vi "Graphics-Init X-axis Overlay.vi"(0 "Ctl Refnum":refnum<vi>, 7 "X-axis slider":refnum<vi>, 11 "error in (no error)":errorcluster) -> (15 "error out":errorcluster)   [LabVIEW 2020]
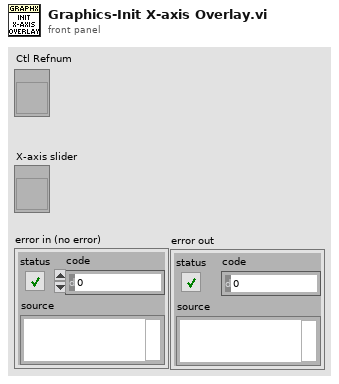
[diagram p1: front panel]
types:
  T1 = typedef "LVRectTypeDef.ctl" = cluster{"Left":i16, "Top":i16, "Right":i16, "Bottom":i16}
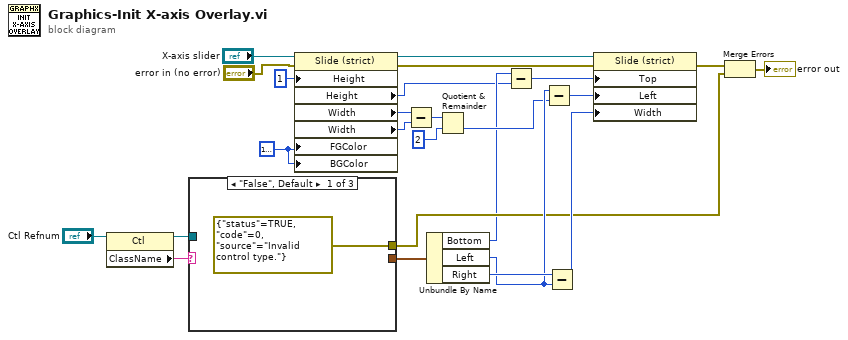
[diagram p0: block diagram]
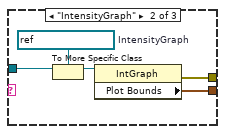
[diagram p2: hidden frame]
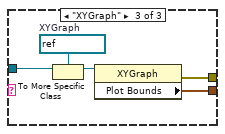
[diagram p3: hidden frame]
diagram:
  w8 = u32 16777216
  n1 = property class="Ctl"(reference="Ctl Refnum") -> (reference out=w5:refnum<vi>, "ClassName"=w6:string)  [unwired: 1 in, 1 out]
  n2 = case shown="\"False\", Default" w6 {
    tunnel: [_ w31 w36] -> w22
    tunnel: [errorcluster {"status"=TRUE, "code"=0, "source"="Invalid control type."} ("error out") w30 w35] -> w10
    tunnel: w5 -> [_ w29 w34]
    frame "False", Default {
    }
    frame "IntensityGraph" {
      w28 = refnum<vi> refnum  # IntensityGraph
      n3 = To More Specific Class(target class=w28, reference=w29) -> (specific class reference=w27:refnum<vi>)  [unwired: 1 in, 1 out]
      n4 = property class="IntGraph"(reference=w27) -> (error out=w30:errorcluster, "Plot Bounds"=w31:T1)  [unwired: 1 in, 1 out]
    }
    frame "XYGraph" {
      w33 = refnum<vi> refnum  # XYGraph
      n5 = To More Specific Class(target class=w33, reference=w34) -> (specific class reference=w32:refnum<vi>)  [unwired: 1 in, 1 out]
      n6 = property class="XYGraph"(reference=w32) -> (error out=w35:errorcluster, "Plot Bounds"=w36:T1)  [unwired: 1 in, 1 out]
    }
  }
  n7 = property class="Slide (strict)"(reference="X-axis slider", error in="error in (no error)", "Height"=u32 1 ("Housing Size:Width"), "FGColor"=w8, "BGColor"=w8) -> (reference out=w23:refnum<vi>, error out=w20:errorcluster, "Height"=w1:u32, "Width"=w19:u32, "Width"=w18:u32)
  n8 = Subtract(x=w19, y=w18) -> (x-y=w17:u32)
  n9 = Unbundle By Name(w22) -> ("Bottom"=w3:i16, "Left"=w14:i16, "Right"=w24:i16)
  n10 = Quotient & Remainder(x=w17, y=u32 2) -> (floor(x/y)=w13:u32)  [unwired: 1 out]
  n11 = Subtract(x=w3, y=w1) -> (x-y=w4:u32)
  n12 = Subtract(x=w14, y=w13) -> (x-y=w15:u32)
  n13 = Subtract(x=w24, y=w14) -> (x-y=w25:i16)
  n14 = property class="Slide (strict)"(reference=w23, error in=w20, "Top"=w4, "Left"=w15, "Width"=w25) -> (error out=w12:errorcluster)  [unwired: 1 out]
  n15 = Merge Errors(w12, w10) -> (→"error out":errorcluster)
